vi "WCA_GET_PHOTOMIXER.vi"(0 "Cartridge Band":u32=10, 1 "Slave Node in":cluster{"Address":i16, "Serial Number":i8[]}={"Address"=19, "Serial Number"=[16, 71, 55, 76, 1, 8, 0, -15]} {"Serial Number" format="%.0x"; "Address" format="%.0x"}, 2 "ObjHandle in":u32, 9 "avg":u32=1, 11 "error in (no error)":errorcluster) -> (4 "ObjHandle out":u32=92930112, 8 "GET_PHOTOMIXER":T1, 15 "error out":errorcluster)   [LabVIEW 2017]
uses:
  WCA_Global.vi
panel:
  # "Node Address"
  # "Serial Number"
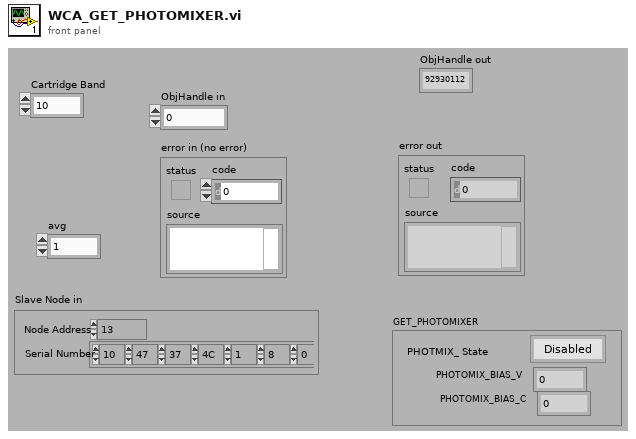
[diagram p1: front panel]
types:
  T1 = cluster{"PHOTMIX_ State":enum16{"Disabled", "Enabled"}, "PHOTOMIX_BIAS_V":sgl, "PHOTOMIX_BIAS_C":sgl}
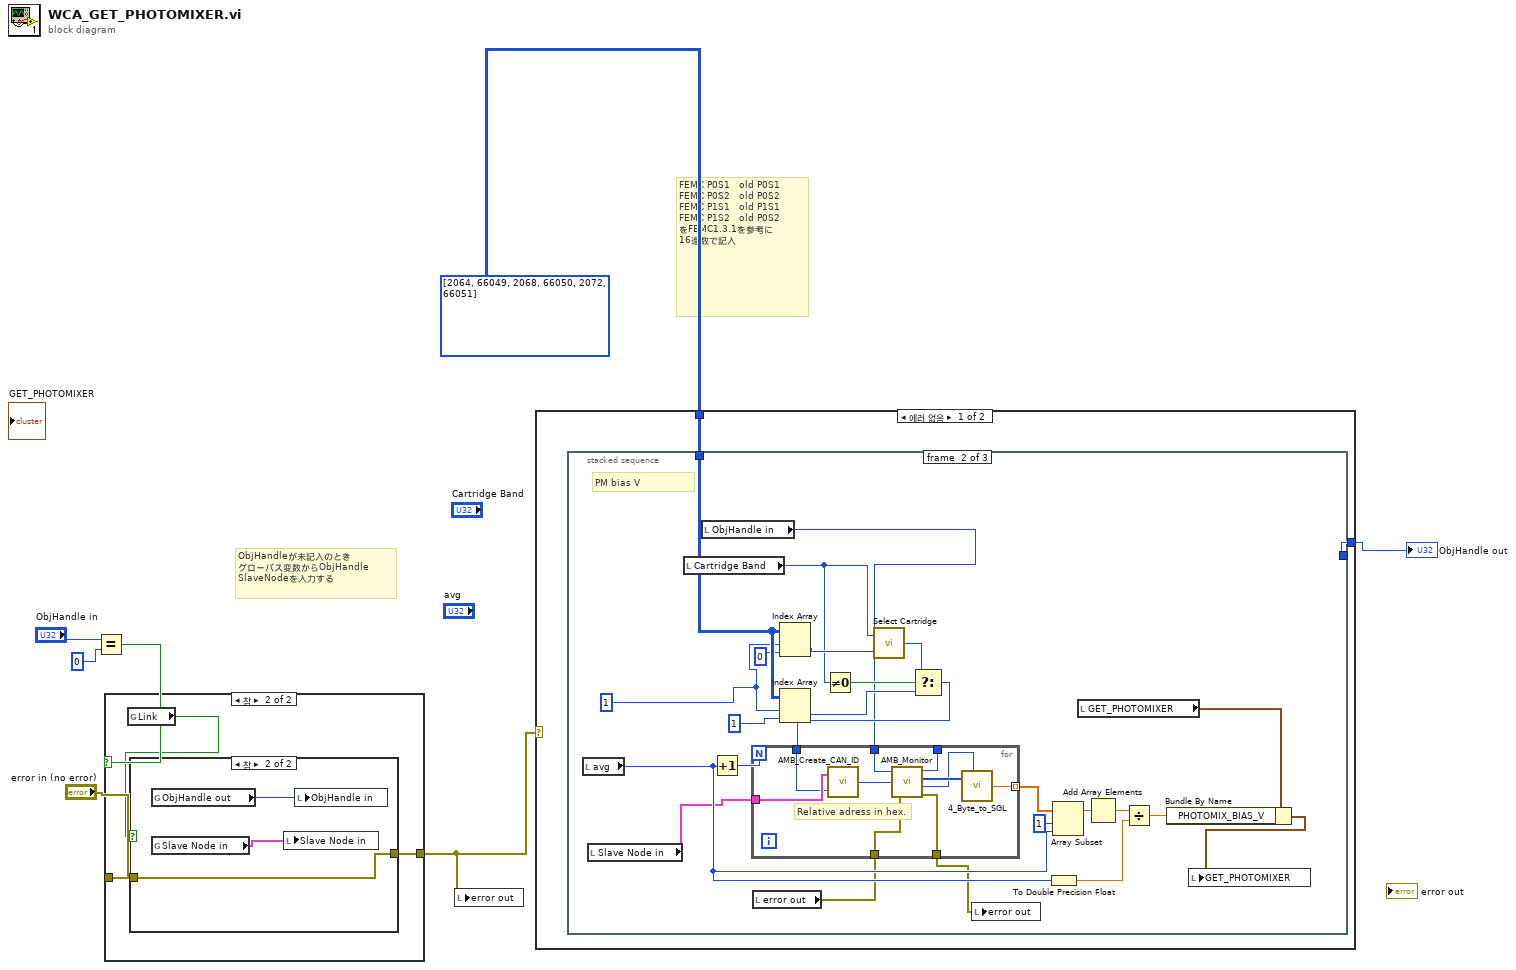
[diagram p0: block diagram]
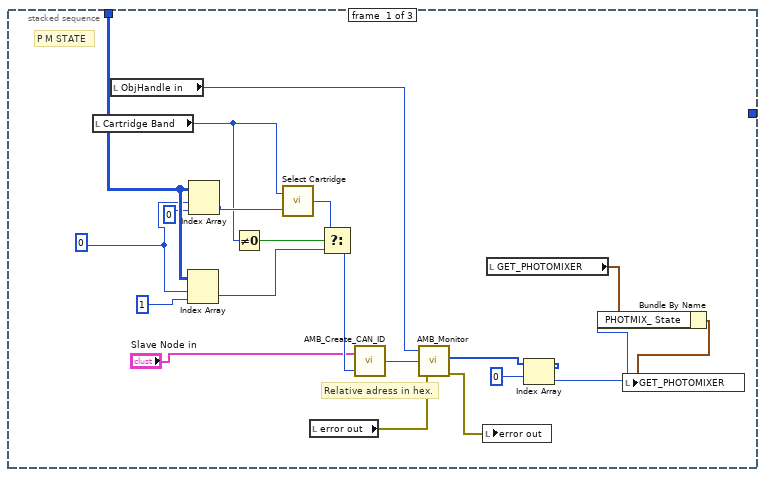
[diagram p2: hidden frame]
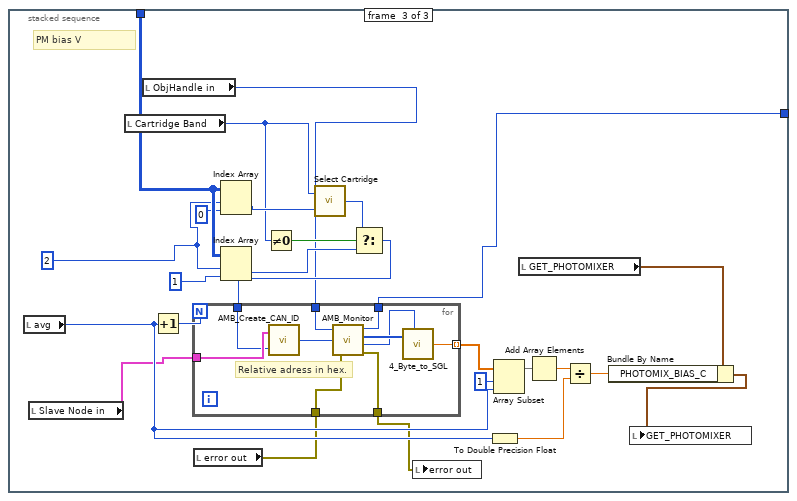
[diagram p3: hidden frame]
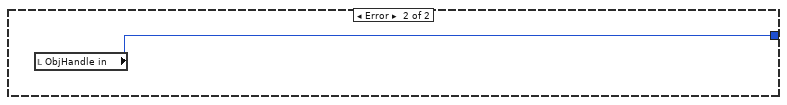
[diagram p4: hidden frame]
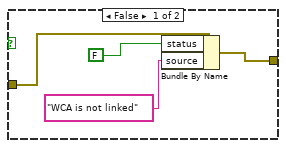
[diagram p6: hidden frame]
diagram:
  # "ObjHandleが未記入のとき\nグローバス変数からObjHandle\nSlaveNodeを入力する"
  # "FEMC P0S1   old P0S1\nFEMC P0S2   old P0S2\nFEMC P1S1   old P1S1\nFEMC P1S2   old P0S2\nをFEMC1.3.1を参考に\n16進数で記入"
  n1 = Equal?(x="ObjHandle in", y=0) -> (x = y?=w5:bool)
  n2 = case shown="참" w5 {
    tunnel: "error in (no error)" -> [w8 w11]
    tunnel: [w8 w10] -> w3
    frame False {
    }
    frame True {
      n3 = global read "WCA_Global.vi" "Link"() -> (w9:bool)
      n4 = case shown="참" w9 {
        tunnel: w11 -> [w15 w16]
        tunnel: [w12 w16] -> w10
        frame False {
          n5 = Bundle By Name(cluster=w15, "status"=FALSE, "source"="WCA is not linked") -> (w12:errorcluster)
        }
        frame True {
          n6 = global read "WCA_Global.vi" "ObjHandle out"() -> (w18:u32)
          n7 = global read "WCA_Global.vi" "Slave Node in"() -> (w17:cluster{"Address":i16, "Serial Number":i8[]})
          n8 = local write "Slave Node in"(w17) -> ()
          n9 = local write "ObjHandle in"(w18) -> ()
        }
      }
    }
  }
  n10 = local write "error out"(w3) -> ()
  n11 = case shown="에러 없음" w3 {
    tunnel: [w19 w110] -> w2
    tunnel: i32[][] [[2064, 66049], [2068, 66050], [2072, 66051]] -> [w20 _]
    frame No Error {
      n12 = stacked-sequence {
        tunnel: w20 -> [w40 w64 w99]
        tunnel: [_ _ w75] -> w19
        frame #0 {
          w21 = 0
          # "Relative adress in hex."
          # "P M STATE"
          n13 = local read "Cartridge Band"() -> (w22:u32)
          n14 = local read "ObjHandle in"() -> (w35:u32)
          n15 = Index Array(array=w40, index (row)=w21, index (col)=1) -> (element=w34:i32)
          n16 = Index Array(array=w40, index (row)=w21, index (col)=0) -> (element=w33:i32)
          n17 = Not Equal To 0?(x=w22) -> (x != 0?=w37:bool)
          n18 = call "Select Cartridge.vi"("Relative Address in"=w33, "Cartridge band"=w22) -> ("Relative Address out"=w38:u32)
          n19 = local read "error out"() -> (w24:errorcluster)
          n20 = Select(t=w38, s=w37, f=w34) -> (s? t:f=w39:u32)
          n21 = call "AMB_Create_CAN_ID.vi"("Relative Address in"=w39, "Slave Node in"="Slave Node in") -> ("CAN ID out"=w30:u32)
          n22 = call "AMB_Monitor.vi"("ObjHandle in"=w35, "CAN ID in"=w30, "error in"=w24) -> ("Data Array out"=w29:u8[], "error out"=w23:errorcluster)  [unwired: 2 out]
          n23 = local write "error out"(w23) -> ()
          n24 = local read "GET_PHOTOMIXER"() -> (w27:T1)
          n25 = Index Array(array=w29, index=0) -> (element=w26:u8)
          n26 = Bundle By Name(cluster=w27, "PHOTMIX_ State"=w26) -> (w25:T1)
          n27 = local write "GET_PHOTOMIXER"(w25) -> ()
        }
        frame #1 {
          w41 = 1
          # "PM bias V"
          n28 = local read "avg"() -> (w48:u32)
          n29 = local read "Slave Node in"() -> (w42:cluster{"Address":i16, "Serial Number":i8[]})
          n30 = local read "Cartridge Band"() -> (w55:u32)
          n31 = local read "ObjHandle in"() -> (w46:u32)
          n32 = Increment(x=w48) -> (x+1=w50:u32)
          n33 = local read "error out"() -> (w44:errorcluster)
          n34 = Index Array(array=w64, index (row)=w41, index (col)=0) -> (element=w60:i32)
          n35 = Index Array(array=w64, index (row)=w41, index (col)=1) -> (element=w61:i32)
          n36 = Not Equal To 0?(x=w55) -> (x != 0?=w62:bool)
          n37 = call "Select Cartridge.vi"("Relative Address in"=w60, "Cartridge band"=w55) -> ("Relative Address out"=w63:u32)
          n38 = Select(t=w63, s=w62, f=w61) -> (s? t:f=w47:u32)
          n39 = for {
            N: w50 -> [_]
            tunnel: [w73] -> _
            tunnel: [w72] -> w43
            tunnel: [w70] -> w51 mode=indexing
            tunnel: w42 -> [w68]
            tunnel: w47 -> [w67]
            tunnel: w46 -> [w66]
            tunnel: w44 -> [w65]
            # "Relative adress in hex."
            n40 = call "AMB_Create_CAN_ID.vi"("Relative Address in"=w67, "Slave Node in"=w68) -> ("CAN ID out"=w74:u32)
            n41 = call "AMB_Monitor.vi"("ObjHandle in"=w66, "CAN ID in"=w74, "error in"=w65) -> ("ObjHandle out"=w73:u32, "Data Array out"=w71:u8[], "Data Length out"=w69:u8, "error out"=w72:errorcluster)
            n42 = call "4_Byte_to_SGL.vi"("Array of 4 bytes"=w71, "number of valid bytes"=w69) -> ("Number"=w70:sgl)  [unwired: 1 out]
          }
          n43 = local write "error out"(w43) -> ()
          n44 = To Double Precision Float(number=w48) -> (double precision float=w49:dbl)
          n45 = Array Subset(array=w51, index=1, length=w48) -> (w53:sgl[])
          n46 = local read "GET_PHOTOMIXER"() -> (w57:T1)
          n47 = Add Array Elements(numeric array=w53) -> (sum=w54:sgl)
          n48 = Divide(x=w54, y=w49) -> (x/y=w45:dbl)
          n49 = Bundle By Name(cluster=w57, "PHOTOMIX_BIAS_V"=w45) -> (w56:T1)
          n50 = local write "GET_PHOTOMIXER"(w56) -> ()
        }
        frame #2 {
          w76 = 2
          # "PM bias V"
          n51 = local read "avg"() -> (w83:u32)
          n52 = local read "Slave Node in"() -> (w77:cluster{"Address":i16, "Serial Number":i8[]})
          n53 = local read "Cartridge Band"() -> (w90:u32)
          n54 = local read "ObjHandle in"() -> (w81:u32)
          n55 = Increment(x=w83) -> (x+1=w85:u32)
          n56 = local read "error out"() -> (w79:errorcluster)
          n57 = Index Array(array=w99, index (row)=w76, index (col)=0) -> (element=w95:i32)
          n58 = Index Array(array=w99, index (row)=w76, index (col)=1) -> (element=w96:i32)
          n59 = Not Equal To 0?(x=w90) -> (x != 0?=w97:bool)
          n60 = call "Select Cartridge.vi"("Relative Address in"=w95, "Cartridge band"=w90) -> ("Relative Address out"=w98:u32)
          n61 = Select(t=w98, s=w97, f=w96) -> (s? t:f=w82:u32)
          n62 = for {
            N: w85 -> [_]
            tunnel: [w108] -> w75
            tunnel: [w107] -> w78
            tunnel: [w105] -> w86 mode=indexing
            tunnel: w77 -> [w103]
            tunnel: w82 -> [w102]
            tunnel: w81 -> [w101]
            tunnel: w79 -> [w100]
            # "Relative adress in hex."
            n63 = call "AMB_Create_CAN_ID.vi"("Relative Address in"=w102, "Slave Node in"=w103) -> ("CAN ID out"=w109:u32)
            n64 = call "AMB_Monitor.vi"("ObjHandle in"=w101, "CAN ID in"=w109, "error in"=w100) -> ("ObjHandle out"=w108:u32, "Data Array out"=w106:u8[], "Data Length out"=w104:u8, "error out"=w107:errorcluster)
            n65 = call "4_Byte_to_SGL.vi"("Array of 4 bytes"=w106, "number of valid bytes"=w104) -> ("Number"=w105:sgl)  [unwired: 1 out]
          }
          n66 = local write "error out"(w78) -> ()
          n67 = To Double Precision Float(number=w83) -> (double precision float=w84:dbl)
          n68 = Array Subset(array=w86, index=1, length=w83) -> (w88:sgl[])
          n69 = local read "GET_PHOTOMIXER"() -> (w92:T1)
          n70 = Add Array Elements(numeric array=w88) -> (sum=w89:sgl)
          n71 = Divide(x=w89, y=w84) -> (x/y=w80:dbl)
          n72 = Bundle By Name(cluster=w92, "PHOTOMIX_BIAS_C"=w80) -> (w91:T1)
          n73 = local write "GET_PHOTOMIXER"(w91) -> ()
        }
      }
    }
    frame Error {
      n74 = local read "ObjHandle in"() -> (w110:u32)
    }
  }
  "ObjHandle out" <- w2
